vi "ReadPCCamera.vi"(2 "error in (no error)":errorcluster, 3 "Camera Reference":i64) -> (0 "error out":errorcluster, 1 "PC Image Out":T1 {"Dialogs" format="%.0b"})   [LabVIEW 2022 SP3]
uses:
  <vilib>/addons/RoboLab/ImageProcessing/QTLIB_2595_LV86/QT_Image.ctl
  <vilib>/addons/RoboLab/ImageProcessing/WindowsDriver/LVDS.dll
panel:
  in  "PC Image":T1={"Width"=640, "Height"=480, "Depth"=32, "data"=[], "Compressed data"=[], "Color table"=[], "Duration"=0, "Options"=0, "Timestamp"=0, "ID"=0, "Reserved"=0, "Dialogs"=0} {"Dialogs" format="%.0b"}
  out "buffersize":i32
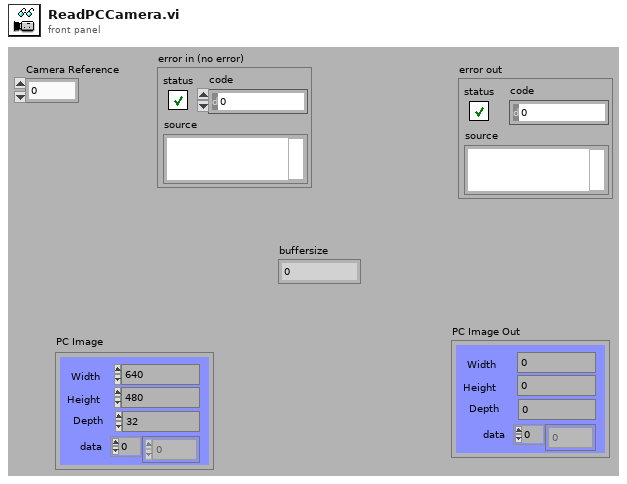
[diagram p1: front panel]
types:
  T1 = typedef "QT_Image.ctl" = cluster{"Width":i32, "Height":i32, "Depth":i32, "data":u8[], "Compressed data":u8[], "Color table":u32[], "Duration":i32, "Options":i32, "Timestamp":i32, "ID":i32, "Reserved":i32, "Dialogs":u32}
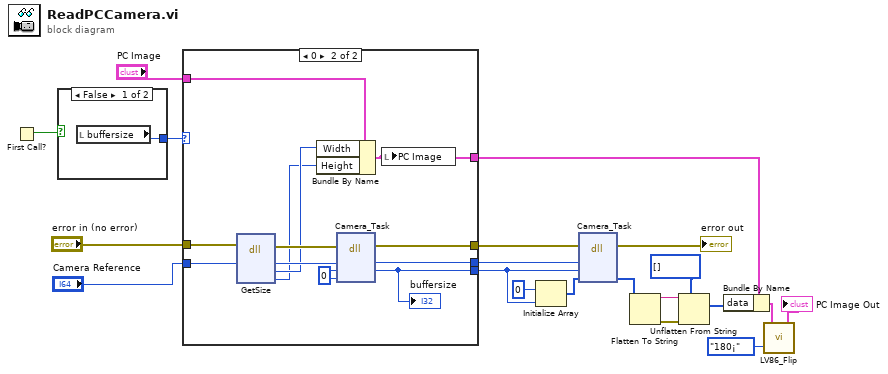
[diagram p0: block diagram]
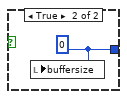
[diagram p2: hidden frame]
diagram:
  n1 = First Call?() -> (First Call?: T/F=w5:bool)
  n2 = case shown="False" w5 {
    tunnel: [w21 w22] -> w4
    frame False {
      n3 = local read "buffersize"() -> (w21:i32)
    }
    frame True {
      w22 = 0
      n4 = local write "buffersize"(w22) -> ()
    }
  }
  n5 = case shown="0" w4 {
    selector: w4 -> [w24 _]
    tunnel: "error in (no error)" -> [w26 w38]
    tunnel: [w26 w37] -> w10
    tunnel: [w23 w36] -> w11
    tunnel: [w25 w27] -> w12
    tunnel: [w24 w35] -> w18
    tunnel: "PC Image" -> [w25 w29]
    tunnel: "Camera Reference" -> [w23 w28]
    frame Default {
    }
    frame 0 {
      w30 = 0 ("buffersize")
      n6 = dll-call lib="C:/Program Files (x86)/National Instruments/LabVIEW 2022/vi.lib/addons/RoboLab/ImageProcessing/WindowsDriver/LVDS.dll" fn="GetSize"(error in=w38, "cameraReference"=w28) -> (error out=w33:errorcluster, "cameraReference"=w34:i64, "width"=w32:i32, "height"=w31:i32)  [unwired: 5 in, 1 out]
      n7 = Bundle By Name(cluster=w29, "Width"=w32, "Height"=w31) -> (w27:T1)
      n8 = dll-call lib="C:/Program Files (x86)/National Instruments/LabVIEW 2022/vi.lib/addons/RoboLab/ImageProcessing/WindowsDriver/LVDS.dll" fn="Camera_Task"(error in=w33, "cameraReference"=w34, "buffersize"=w30, "Buffer"=w30) -> (error out=w37:errorcluster, "cameraReference"=w36:i64, "buffersize"=w35:i32)  [unwired: 4 in, 1 out]
      "buffersize" <- w35
      n9 = local write "PC Image"(w27) -> ()
    }
  }
  n10 = Initialize Array(0 ("Buffer"), w18) -> (w8:i32[])
  n11 = dll-call lib="C:/Program Files (x86)/National Instruments/LabVIEW 2022/vi.lib/addons/RoboLab/ImageProcessing/WindowsDriver/LVDS.dll" fn="Camera_Task"(error in=w10, "cameraReference"=w11, "buffersize"=w18, "Buffer"=w8) -> (error out=→"error out":errorcluster, "Buffer"=w13:i32[])  [unwired: 5 in, 1 out]
  n12 = Flatten To String(anything=w13) -> (data string=w15:string, error out=w14:errorcluster)  [unwired: 3 in, 1 out]
  n13 = Unflatten From String(type=u8[] [], binary string=w15, error in (no error)=w14) -> (value=w16:u8[])  [unwired: 2 in, 2 out]
  n14 = Bundle By Name(cluster=w12, "data"=w16) -> (w3:T1)
  n15 = call <vilib>:"LV86_Flip.vi"("Flip"=enum16{"90¡", "180¡", "270¡"}."180¡", "Image"=w3) -> ("Image"=→"PC Image Out":T1)  [unwired: 1 in]
